vi "Get Install Path From Source Path.vi"(8 "Error In":errorcluster, 10 "Source File Path":path, 11 "Configuration":T1) -> (0 "Error Out":errorcluster, 1 "Relative File Path":string, 2 "Install File Path":path, 3 "Configuration":T1)   [LabVIEW 2011, in "LVH-Build-Tools.lvlib"]
doc: "Get the install path of a file or folder from its source path.\n\nThis VI strips the source root path from the file path and prepends the install path."
uses:
  LVH-Build-Tools.lvlib
  Type Defs/Configuration.ctl
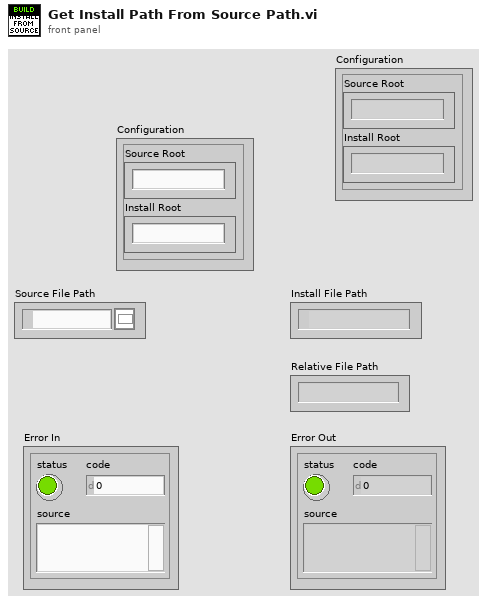
[diagram p1: front panel]
types:
  T1 = typedef "LVH-Build-Tools.lvlib/Configuration.ctl" = cluster{"Source Root":string, "Install Root":string, "Components":string[], "Ignore":string[]}
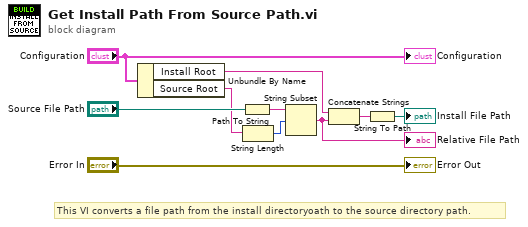
[diagram p0: block diagram]
diagram:
  # "This VI converts a file path from the install directoryoath to the source directory path."
  n1 = Unbundle By Name("Configuration") -> ("Install Root"=w2:string, "Source Root"=w3:string)
  n2 = Path To String(path="Source File Path") -> (string=w9:string)
  n3 = String Length(string=w3) -> (length=w10:i32)
  n4 = String Subset(string=w9, offset (0)=w10) -> (substring=w4:string)  [unwired: 1 in]
  "Relative File Path" <- w4
  n5 = Concatenate Strings(w2, w4) -> (w6:string)
  n6 = String To Path(string=w6) -> (path=→"Install File Path":path)
  "Error Out" <- "Error In"
  "Configuration" <- "Configuration"
